vi "Create.vi"(8 "error in (no error)":errorcluster, 11 "IP Address and Port":string) -> (0 "error out":errorcluster, 3 "Connection out":refnum<class "Connection.lvclass">)   [LabVIEW 2010, in "MDSplus.lvlib" / "Connection.lvclass"]
uses:
  <vilib>/MDSplus/Classes/Connection_Class/Connection.lvclass
  <vilib>/MDSplus/Classes/Connection_Class/Connection.lvclass/Connection.ctl
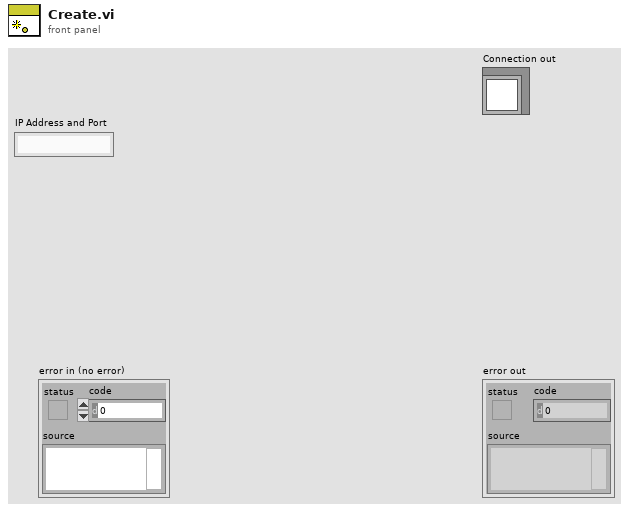
[diagram p1: front panel]
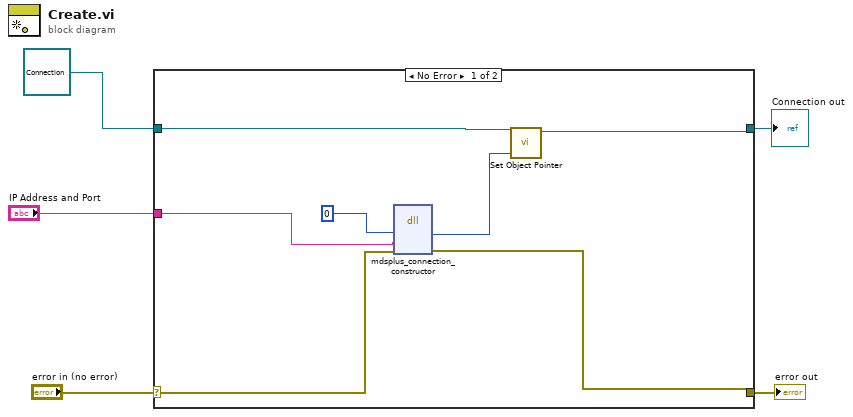
[diagram p0: block diagram]
diagram:
  n1 = case shown="No Error" "error in (no error)" {
    selector: "error in (no error)" -> [w10 w14]
    tunnel: [w9 w14] -> w4
    tunnel: [w7 w13] -> w2
    tunnel: refnum<class "Connection.lvclass"> refnum ("Connection in") -> [w8 w13]
    tunnel: "IP Address and Port" -> [w11 _]
    frame No Error {
      n2 = dll-call lib="MDSobjectsLVShr" fn="mdsplus_connection_constructor"("lvEventPtr"=i64 0 ("lvTreePtr"), "evNameIn"=w11, "error"=w10) -> ("lvEventPtr"=w6:i64, "error"=w9:errorcluster)  [unwired: 5 in, 2 out]
      n3 = call <vilib>:"Set Object Pointer.vi"("Object Pointer"=w6, "Connection in"=w8) -> ("Connection out"=w7:refnum<class "Connection.lvclass">)  [unwired: 8 in, 1 out]
    }
    frame Error {
    }
  }
  "error out" <- w4
  "Connection out" <- w2
